vi "Test Setup Error.vi"(8 "error in (no error)":errorcluster, 11 "Error Checking Test in":refnum<class "Error Checking Test.lvclass">) -> (0 "error out":errorcluster, 3 "Error Checking Test out":refnum<class "Error Checking Test.lvclass">)   [LabVIEW 2020, in "Error Checking Test.lvclass"]
uses:
  Error Checking Test.lvclass
  Error Checking Test.lvclass/Error Checking Test.ctl
  LUnit Test Case/LUnit Test Case V2.lvclass
  Result/Status.ctl
  Result/Result.lvlib
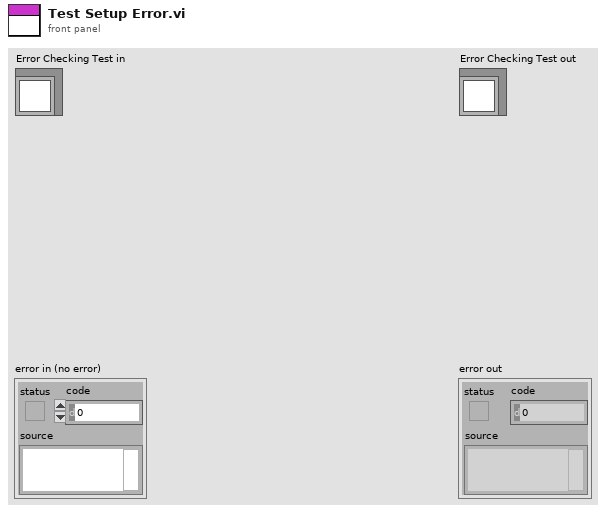
[diagram p1: front panel]
types:
  T1 = typedef "Result.lvlib/Status.ctl" = enum16{"", "Passed", "Failed", "Error", "Skipped", "Setup Error", "Broken", "Teardown Error"}
  T2 = typedef "Result.lvlib/Result.ctl" = cluster{"Name":string, "Message":string, "Description":string, "Status":T1, "Result Type":T3, "Execution Time":dbl}
  T3 = typedef "Result.lvlib/Type.ctl" = enum16{"Method", "Case", "Suite", "Pass", "Fail", "Skip", "Pass if", "Fail if", "Pass if Error", "Fail if Error", "Pass if Equal", "Fail if Equal"}
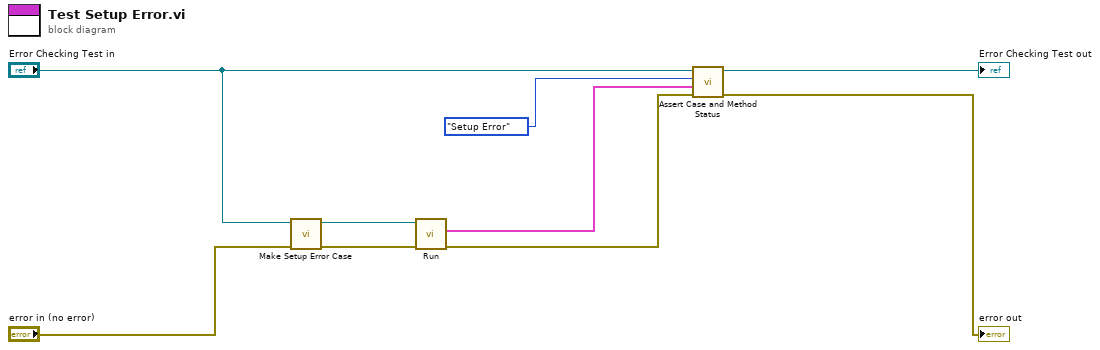
[diagram p0: block diagram]
diagram:
  n1 = call "Make Setup Error Case.vi"("error in (no error)"="error in (no error)", "Error Checking Test in"="Error Checking Test in") -> ("error out"=w5:errorcluster, "LUnit Test Case V2 out"=w6:refnum<class "LUnit Test Case V2.lvclass">)  [unwired: 8 in]
  n2 = call-dynamic "Run.vi"("error in (no error)"=w5, "LUnit Test Case V2 in"=w6) -> ("error out"=w3:errorcluster, "Results"=w2:T2[])  [unwired: 8 in]
  n3 = call "Assert Case and Method Status.vi"("error in (no error)"=w3, "Results"=w2, "Status"=Status."Setup Error", "Error Checking Test in"="Error Checking Test in") -> ("error out"=→"error out":errorcluster, "Error Checking Test out"=→"Error Checking Test out":refnum<class "Error Checking Test.lvclass">)  [unwired: 6 in]
